vi "Configure Harmonics Group.vi"(8 "error in (no error)":errorcluster, 9 "Group (1: Harmonics 1)":i32(ring)=1 items=["Harmonics 1"=1, "Harmonics 2"=2], 10 "Element/Wiring Unit (0: ALL)":i32(ring) items=["All", "1", "2", "3", "4", "5", "6", "Sigma A", "Sigma B", "Sigma C"], 11 "VISA resource name":refnum<visa-resource-name>) -> (0 "error out":errorcluster, 3 "VISA resource name out":refnum<visa-resource-name>)   [LabVIEW 2021, in "Yokogawa WT1800 Series.lvlib"]
doc: "Configures the harmonics group features.\nYou can divide all the input elements into two groups: Haromics 1 and Haromics 2, and measure harmonics using two PLL sources with different frequencies. You can measure the input and output harmonics of an AC.AC converter whose input and output frequencies are different.\n\n<b>Note:</b>\nThis setting valid on models with the simultaneous dual harmonic measurement (/G6) option."
uses:
  <instrlib>/Yokogawa WT1800 Series/Yokogawa WT1800 Series.lvlib
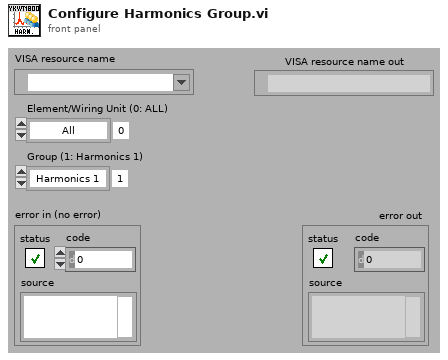
[diagram p1: front panel]
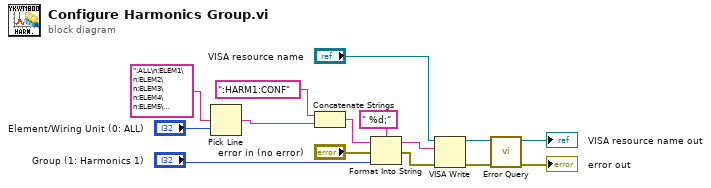
[diagram p0: block diagram]
diagram:
  n1 = Pick Line ("ライン選択")(multi-line string=":ALL\n:ELEM1\n:ELEM2\n:ELEM3\n:ELEM4\n:ELEM5\n:ELEM6\n:SIGMA\n:SIGMB\n:SIGMC" ("複数行文字列"), line index="Element/Wiring Unit (0: ALL)") -> (output string=w5:string)  [unwired: 1 in]
  n2 = Concatenate Strings(":HARM1:CONF", w5) -> (w3:string)
  n3 = Format Into String ("文字列にフォーマット")(format string=" %d;" ("形式文字列"), initial string=w3, error in="error in (no error)", "Group (1: Harmonics 1)") -> (resulting string=w8:string, error out=w9:errorcluster)
  n4 = VISA Write ("VISA書き込み")(VISA resource name="VISA resource name", write buffer=w8, error in (no error)=w9) -> (VISA resource name out=w15:refnum<visa-resource-name>, error out=w14:errorcluster)  [unwired: 1 out]
  n5 = call <instrlib>:"Error Query.vi"("error in (no error)"=w14, "VISA resource name"=w15) -> ("error out"=→"error out":errorcluster, "VISA resource name out"=→"VISA resource name out":refnum<visa-resource-name>)  [unwired: 6 in, 2 out]
